vi "Read Config.vi"(8 "error in (no error)":errorcluster, 9 "Re-Init?":bool, 10 "ICM File In":path, 11 "Multi Parser in":refnum<class "Mulit Sentence Parser.lvclass">) -> (0 "error out":errorcluster, 3 "Multi Parser out":refnum<class "Mulit Sentence Parser.lvclass">)   [LabVIEW 2015, in "Mulit Sentence Parser.lvclass"]
doc: "Multi Sentencel Parser.lvclass:Read Config.vi\n\nThis VI reads the Multi Sentence Parser Class parameters from the ICM configuration file.\n\nInstrument Communication Module Version 1.0\nOctober, 2018 Original Code Consulting David Thomson\n www.originalcode.com"
uses:
  Mulit Sentence Parser.lvclass
  Mulit Sentence Parser.lvclass/Mulit Sentence Parser.ctl
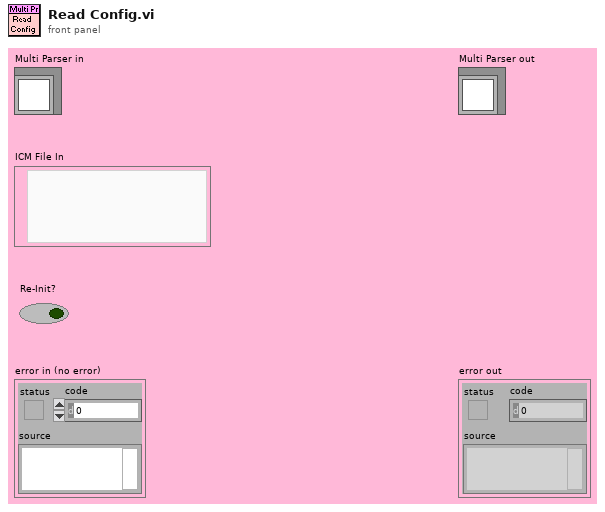
[diagram p1: front panel]
types:
  T1 = typedef "Mulit Sentence Parser.lvclass/Multi Sentence Parser Config.ctl" = cluster{"Sentences":cluster{"Sentence ID":string, "Format String":string, "Channels":string[], "Enabled":bool[]}[]}
  T2 = cluster{"Sentence ID":string, "Format String":string, "Channels":string[], "Enabled":bool[]}[]
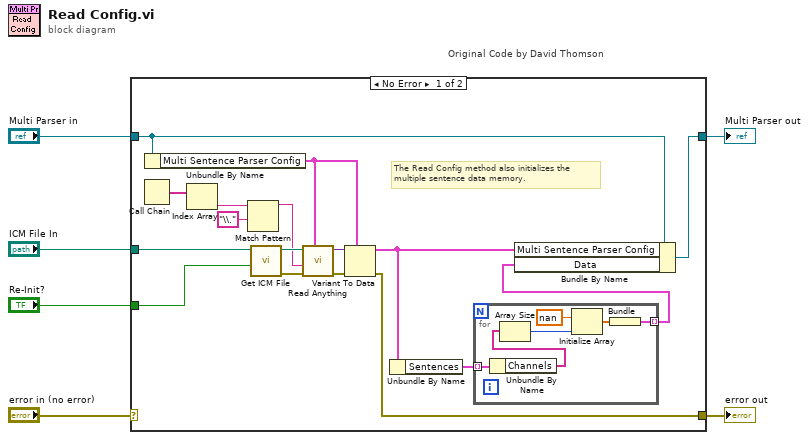
[diagram p0: block diagram]
diagram:
  n1 = case "Original Code by David Thomson" shown="No Error" "error in (no error)" {
    selector: "error in (no error)" -> [_ w31]
    tunnel: [w15 w31] -> w5
    tunnel: [w13 w30] -> w3
    tunnel: "Multi Parser in" -> [w10 w30]
    tunnel: "ICM File In" -> [w12 _]
    tunnel: "Re-Init?" -> [w11 _]
    frame No Error {
      # "The Read Config method also initializes the\nmultiple sentence data memory."
      n2 = Call Chain() -> (call chain=w20:string[])
      n3 = Unbundle By Name(w10) -> ("Multi Sentence Parser Config"=w14:T1)
      n4 = Index Array(array=w20) -> (element=w21:string)  [unwired: 1 in]
      n5 = Match Pattern(string=w21, regular expression="\\.") -> (before substring=w18:string)  [unwired: 1 in, 3 out]
      n6 = call "Get ICM File.vi"("Re-Init?"=w11, "ICM File In"=w12) -> ("error out"=w22:errorcluster, "ICM File"=w23:path)  [unwired: 8 in]
      n7 = call "Read Anything.vi"("Type of Anything"=w14, "Error In"=w22, "Section Name (Name of \"Type of Anything\")"=w18, "Path (dialog)"=w23) -> ("Error Out"=w16:errorcluster, "Anything"=w17:variant)  [unwired: 5 in, 1 out]
      n8 = Variant To Data(error in=w16, type=w14, Variant=w17) -> (data=w9:T1, error out=w15:errorcluster)
      n9 = Unbundle By Name(w9) -> ("Sentences"=w8:T2)
      n10 = for {
        tunnel: w8 -> [w29] mode=indexing
        tunnel: [w24] -> w7 mode=indexing
        n11 = Unbundle By Name(w29) -> ("Channels"=w28:string[])
        n12 = Array Size(array=w28) -> (size(s)=w27:i32)
        n13 = Initialize Array(nan ("element"), w27) -> (w25:dbl[])
        n14 = Bundle(w25) -> (w24:cluster{dbl[]})  [unwired: 1 in]
      }
      n15 = Bundle By Name(cluster=w10, "Multi Sentence Parser Config"=w9, "Data"=w7) -> (w13:refnum<class "Mulit Sentence Parser.lvclass">)
    }
    frame Error {
    }
  }
  "error out" <- w5
  "Multi Parser out" <- w3
